vi "Create.vi"(8 "error in (no error)":errorcluster, 10 "Tests":string[](array[string])) -> (0 "error out":errorcluster, 3 "Static Filter":refnum<class "Filter.lvclass">)   [LabVIEW 2020, in "Static Filter.lvclass"]
uses:
  Static Filter.lvclass
  Filter/Filter.lvclass
  C:/git/astemes-lunit/source/Support/Filters/Filter/Filter.lvclass
  Static Filter.lvclass/Static Filter.ctl
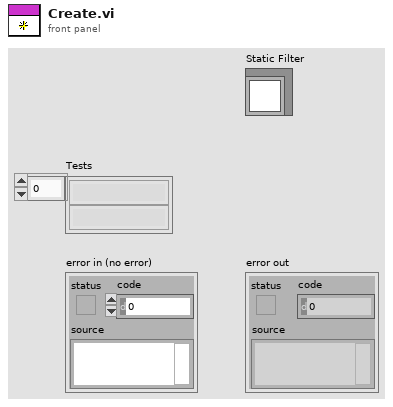
[diagram p1: front panel]
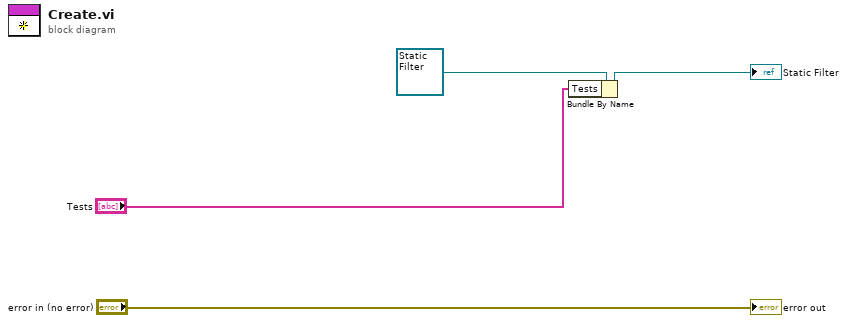
[diagram p0: block diagram]
diagram:
  n1 = Bundle By Name(cluster=refnum<class "Static Filter.lvclass"> refnum ("Static Filter"), "Tests"="Tests") -> (→"Static Filter":refnum<class "Static Filter.lvclass">)
  "error out" <- "error in (no error)"
